vi "Z Go.vi"(8 "error in (no error)":errorcluster, 9 "Speed In":dbl format="%#_13g", 10 "Position In":dbl format="%#_13g", 11 "Gantry":refnum<k24>) -> (0 "error out":errorcluster, 1 "Speed Out":dbl, 2 "Position Out":dbl, 3 "Gantry":refnum<k24>)   [LabVIEW 2020, in "A3200.lvclass"]
uses:
  A3200.lvclass
  C:/Program Files (x86)/Aerotech/A3200/LabVIEW/2010/Bin/Aerotech.A3200.dll
  Program Files (x86)/Aerotech/A3200/LabVIEW/2010/Bin/Aerotech.A3200.dll
  Program Files (x86)/Aerotech/A3200/LabVIEW/2010/Motion/MoveIncSingle.vi
  Aerotech.lvlib
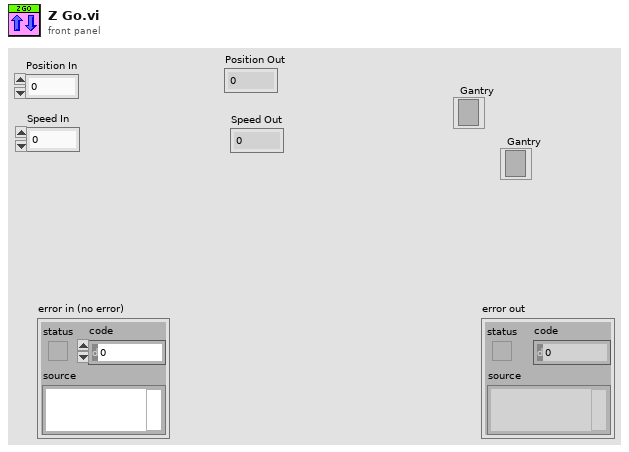
[diagram p1: front panel]
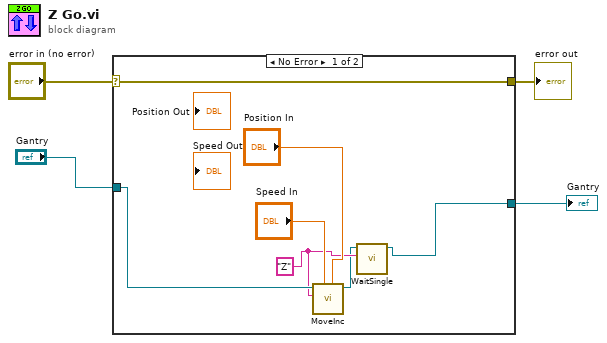
[diagram p0: block diagram]
diagram:
  n1 = case shown="No Error" "error in (no error)" {
    selector: "error in (no error)" -> [w11 w12]
    tunnel: [w11 w12] -> w3
    tunnel: "Gantry" -> [w9 _]
    tunnel: [w10 _] -> w1
    frame No Error {
      w6 = "Z"
      n2 = call-poly "MoveInc.vi"("distance"="Position In", "speed"="Speed In", "axis name"=w6, "controller in"=w9) -> ("controller out"=w5:refnum<k24>)  [unwired: 6 in, 1 out]
      n3 = call "WaitSingle.vi"("axis name"=w6, "controller in"=w5) -> ("controller out"=w10:refnum<k24>)  [unwired: 7 in, 2 out]
    }
    frame Error {
    }
  }
  "error out" <- w3
  "Gantry" <- w1
